vi "Read Settings.vi"(0 "Path":path=path "C:/Users/Kåre Juul Kirkegaard/AppData/Local/Event Diplom/Event2019/settings.ini", 11 "Error in":errorcluster caption="Error in (no error)") -> (4 "Description":string, 15 "Error out":errorcluster)   [LabVIEW 2019]
doc: "<Developer>\nGPower\n10/6 2019"
uses:
  <vilib>/Utility/config.llb/Read Key (String).vi
  <vilib>/Utility/config.llb/NI_LVConfig.lvlib
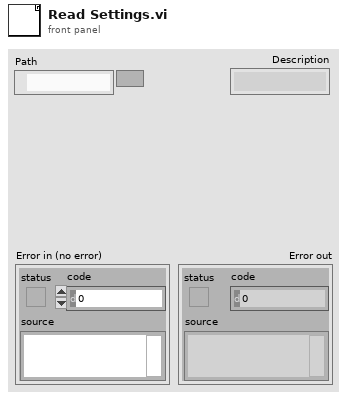
[diagram p1: front panel]
types:
  T1 = typedef "NI_LVConfig.lvlib/Config Data RefNum.ctl" = refnum<k1>
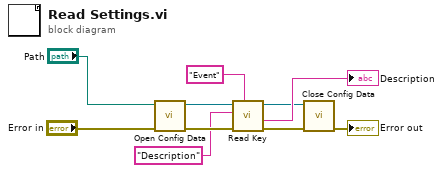
[diagram p0: block diagram]
diagram:
  n1 = call <vilib>:"Open Config Data.vi"("error in (no error)"="Error in", "configuration file path"="Path") -> ("error out"=w9:errorcluster, "refnum"=w8:T1)  [unwired: 7 in, 1 out]
  n2 = call-poly <vilib>:"Read Key.vi"("section"="Event", "error in (no error)"=w9, "key"="Description", "refnum"=w8) -> ("error out"=w5:errorcluster, "value"=→"Description":string, "refnum out"=w3:T1)  [unwired: 4 in, 1 out]
  n3 = call <vilib>:"Close Config Data.vi"("error in (no error)"=w5, "refnum"=w3) -> ("error out"=→"Error out":errorcluster)  [unwired: 8 in, 1 out]
